vi "ShootAngle_Vel.vi"() -> (2 "angle":dbl, 3 "velocity":dbl)   [LabVIEW 2019]
uses:
  Robot Global Data.vi
panel:
  out "vox":dbl
  out "time of flight":dbl
  out "voy":dbl
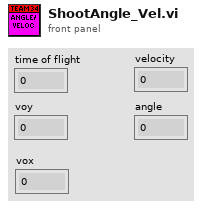
[diagram p1: front panel]
types:
  T1 = typedef "Vision Data.ctl" = cluster{"xOffset":dbl, "yOffset":dbl, "area":dbl, "skewOffset":dbl, "hasTarget":dbl}
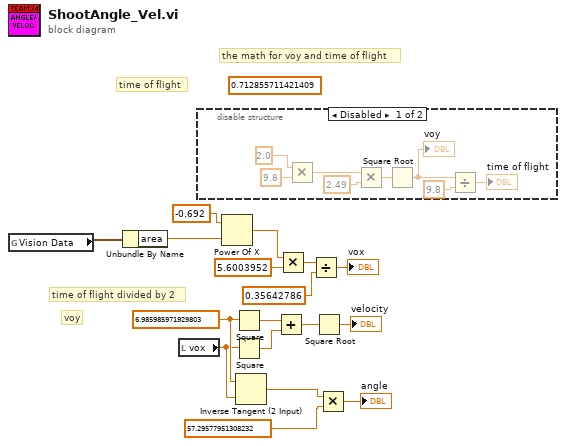
[diagram p0: block diagram]
diagram:
  (unwired) 0.712855711421409
  w13 = 6.985985971929803
  # "time of flight divided by 2"
  # "voy"
  # "time of flight"
  # "the math for voy and time of flight"
  n1 = global read "Robot Global Data.vi" "Vision Data"() -> (w6:T1)
  n2 = Unbundle By Name(w6) -> ("area"=w5:dbl)
  n3 = local read "vox"() -> (w11:dbl)
  n4 = disable-structure shown="Disabled" {
    frame Disabled {
      n5 = Multiply(x=2.0, y=9.8) -> (x*y=w22:dbl)
      n6 = Multiply(x=w22, y=2.49) -> (x*y=w24:dbl)
      n7 = Square Root(x=w24) -> (sqrt(x)=w25:dbl)
      "voy" <- w25
      n8 = Divide(x=w25, y=9.8) -> (x/y=→"time of flight":dbl)
    }
    frame Enabled {
    }
  }
  n9 = Power Of X(1:w5, 2:-0.692 ("y")) -> (0:w3:dbl)
  n10 = Square(x=w13) -> (x^2=w9:dbl)
  n11 = Square(x=w11) -> (x^2=w10:dbl)
  n12 = Inverse Tangent (2 Input)(1:w11, 2:w13) -> (0:w14:dbl)
  n13 = Add(x=w9, y=w10) -> (x+y=w8:dbl)
  n14 = Multiply(x=w3, y=5.6003952) -> (x*y=w1:dbl)
  n15 = Divide(x=w1, y=0.35642786) -> (x/y=→"vox":dbl)
  n16 = Square Root(x=w8) -> (sqrt(x)=→"velocity":dbl)
  n17 = Multiply(x=w14, y=57.29577951308232) -> (x*y=→"angle":dbl)
